vi "SPD.QEvsPow Meas Const T.vi"(5 "Continue":refnum<vi>, 6 "Temperature index":i32, 7 "Progress":refnum<vi>, 8 "Error In":errorcluster, 10 "TR_Bif Params":T1 {"scale type" items=["Linear", "Logarithmic"]}, 11 "SPD.Stand Ctrl in":T2={"spdDeviceSession"={"spdRef"=0, "connected"=FALSE, "spdName"="", "specification"={"diod case"=enum."default", "type"=enum."Unknown", "frequency"=enum."Unknown"}, "hidSPD.Controller"={"TSet"=0.0, "HV_bias"=0.0, "DDS_stb_code"=0}, "hidSPD.Sturtup Values"={"TSet"=0.0, "HV_bias"=0.0, "DDS_stb_code"=0}}, "DevBSession"={"DevBRef"="", "connected"=FALSE}, "FreqCSession"={"FreqCRef"="", "timeout"=0.0, "Gate"=0.0, "connected"=FALSE}, "8164BSession"={"Connection ID"=refnum, "Connected"=FALSE, "Info"="", "Slots Info"=[]}, "LeCroySession"={"LeCroySession"="", "connected"=FALSE}, "Events"={"DCRTest"=refnum, "Stop"=refnum}, "configFile"={"configFile ref"=refnum, "configFile path"=path "", "equipmentFile ref"=refnum}, "SPD.Meas Grid"={"DateTime"="", "DT"=[], "Insensitivity"=[], "Temprature"=[], "Stb_code"=[], "HV_Bias"=[]}, "SPD.Queues"={"state queue"=refnum}, "Console"=refnum} {"spdDeviceSession"."hidSPD.Sturtup Values"."HV_bias" format="%#_6p, V"; "spdDeviceSession"."hidSPD.Sturtup Values"."TSet" format="%#_6p, DegC"; "spdDeviceSession"."hidSPD.Controller"."HV_bias" format="%#_6p, V"; "spdDeviceSession"."hidSPD.Controller"."TSet" format="%#_6p, DegC"}) -> (0 "Error Out":errorcluster, 1 "pass":bool, 2 "Report":string, 3 "SPD.Stand Ctrl out":T2={"spdDeviceSession"={"spdRef"=0, "connected"=FALSE, "spdName"="", "specification"={"diod case"=enum."default", "type"=enum."Unknown", "frequency"=enum."Unknown"}, "hidSPD.Controller"={"TSet"=0.0, "HV_bias"=0.0, "DDS_stb_code"=0}, "hidSPD.Sturtup Values"={"TSet"=0.0, "HV_bias"=0.0, "DDS_stb_code"=0}}, "DevBSession"={"DevBRef"="", "connected"=FALSE}, "FreqCSession"={"FreqCRef"="", "timeout"=0.0, "Gate"=0.0, "connected"=FALSE}, "8164BSession"={"Connection ID"=refnum, "Connected"=FALSE, "Info"="", "Slots Info"=[]}, "LeCroySession"={"LeCroySession"="", "connected"=FALSE}, "Events"={"DCRTest"=refnum, "Stop"=refnum}, "configFile"={"configFile ref"=refnum, "configFile path"=path "", "equipmentFile ref"=refnum}, "SPD.Meas Grid"={"DateTime"="", "DT"=[], "Insensitivity"=[], "Temprature"=[], "Stb_code"=[], "HV_Bias"=[]}, "SPD.Queues"={"state queue"=refnum}, "Console"=refnum} {"spdDeviceSession"."hidSPD.Sturtup Values"."HV_bias" format="%#_6p, V"; "spdDeviceSession"."hidSPD.Sturtup Values"."TSet" format="%#_6p, DegC"; "spdDeviceSession"."hidSPD.Controller"."HV_bias" format="%#_6p, V"; "spdDeviceSession"."hidSPD.Controller"."TSet" format="%#_6p, DegC"})   [LabVIEW 2018]
uses:
  Instruments/KeySight 8164B/KeySight 8164B LAN InstrLib.lvlib
  typedefs/SPD.QE Strobe_Phase Tune Limits.ctl
  <vilib>/Analysis/NI_AALBase.lvlib
  <vilib>/Analysis/1siggen.llb/Ramp Pattern by Samples.vi
  Instruments/KC705 DevBoard/typedefs/DevB.Session.ctl
  Instruments/KeySight 53230A/typedefs/FreqC.Session.ctl
  Instruments/KeySight 8164B/KeySight 8164B LAN InstrLib/typedefs/KeySight 8164B control.ctl
  Instruments/LeCroy SDA830/typedefs/LeCroy.Session.ctl
  typedefs/SPD.Stand Ctrl.ctl
  typedefs/SPD.Events.ctl
  <vilib>/Utility/config.llb/Config Data RefNum.ctl
  <vilib>/Utility/config.llb/NI_LVConfig.lvlib
  typedefs/SPD.Meas Grid.ctl
  typedefs/SPD.Stand state.ctl
  typedefs/SPD.Queues.ctl
  ConfigFile/SPD.Config File ctrl.ctl
  Instruments/SPD HID Interface/hidSPDLibForLabView/LibVIs/hidSPD Controls/hidSPD Controller.ctl
  Instruments/SPD HID Interface/hidSPDLibForLabView/hidSPDLibForLabView.lvlib
  Instruments/SPD HID Interface/hidSPDLibForLabView/LibVIs/hidSPD Controls/hidSPD Device Session.ctl
  Instruments/SPD HID Interface/hidSPDLibForLabView/LibVIs/hidSPD Controls/hidSPD SPD Type.ctl
  typedefs/SPD.QEvsPower Test Params.ctl
  Instruments/SPD HID Interface/hidSPDLibForLabView/LibVIs/hidSPD Controls/hidSPD SPD Diod Case.ctl
  Instruments/SPD HID Interface/hidSPDLibForLabView/LibVIs/hidSPD Controls/hidSPD.STB Frequency.ctl
  Instruments/SPD HID Interface/hidSPDLibForLabView/LibVIs/hidSPD Controls/hidSPD.SPD specification.ctl
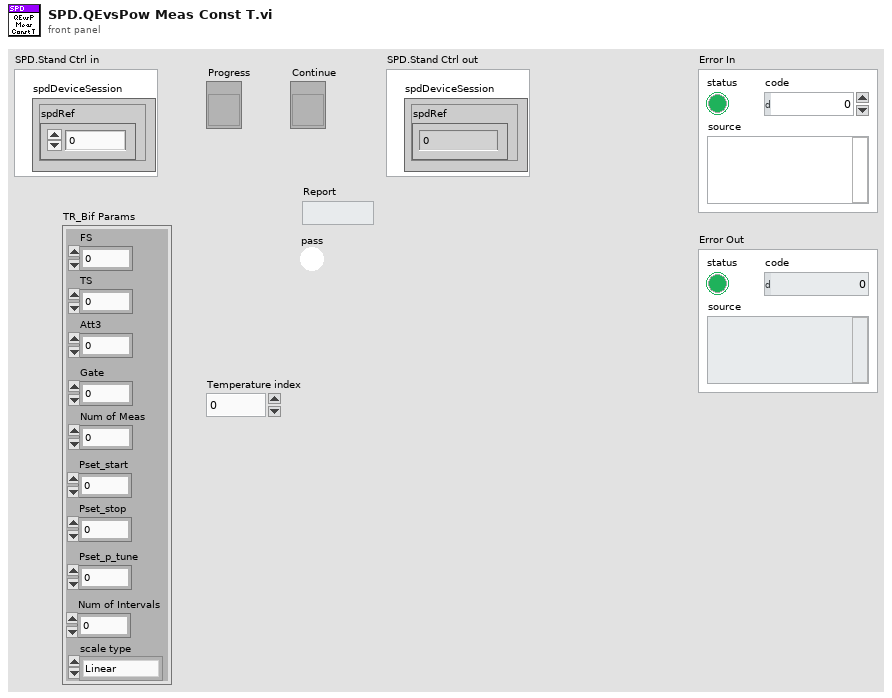
[diagram p1: front panel]
types:
  T1 = typedef "SPD.QEvsPower Test Params.ctl" = cluster{"FS":i32, "TS":i32, "Att3":dbl, "Gate":dbl, "Num of Meas":i32, "Pset_start":dbl, "Pset_p_tune":dbl, "Pset_stop":dbl, "Num of Intervals":i32, "scale type":u16}
  T2 = typedef "SPD.Stand Ctrl.ctl" = cluster{"spdDeviceSession":T3, "DevBSession":T9, "FreqCSession":T10, "8164BSession":T11, "LeCroySession":T12, "Events":T13, "configFile":T14, "SPD.Meas Grid":T16, "SPD.Queues":T17, "Console":refnum<vi>}
  T3 = typedef "hidSPDLibForLabView.lvlib/hidSPD Device Session.ctl" = cluster{"spdRef":u64, "connected":bool, "spdName":string, "specification":T4, "hidSPD.Controller":T8, "hidSPD.Sturtup Values":T8}
  T4 = typedef "hidSPDLibForLabView.lvlib/hidSPD.SPD specification.ctl" = cluster{"diod case":T5, "type":T6, "frequency":T7}
  T5 = typedef "hidSPDLibForLabView.lvlib/hidSPD SPD Diod Case.ctl" = enum16{"Unknown", "default", "butterfly"}
  T6 = typedef "hidSPDLibForLabView.lvlib/hidSPD SPD Type.ctl" = enum16{"Unknown", "Free Run", "Gate"}
  T7 = typedef "hidSPDLibForLabView.lvlib/hidSPD.STB Frequency.ctl" = enum16{"Unknown", "312", "1250"}
  T8 = typedef "hidSPDLibForLabView.lvlib/hidSPD Controller.ctl" = cluster{"TSet":sgl, "HV_bias":sgl, "DDS_stb_code":u16}
  T9 = typedef "DevB.Session.ctl" = cluster{"DevBRef":refnum<visa-resource-name>, "connected":bool}
  T10 = typedef "FreqC.Session.ctl" = cluster{"FreqCRef":refnum<visa-resource-name>, "timeout":dbl, "Gate":dbl, "connected":bool}
  T11 = typedef "KeySight 8164B LAN InstrLib.lvlib/KeySight 8164B control.ctl" = cluster{"Connection ID":refnum<k5>, "Connected":bool, "Info":string, "Slots Info":string[]}
  T12 = typedef "LeCroy.Session.ctl" = cluster{"LeCroySession":refnum<visa-resource-name>, "connected":bool}
  T13 = typedef "SPD.Events.ctl" = cluster{"DCRTest":refnum<user-event>, "Stop":refnum<user-event>}
  T14 = typedef "SPD.Config File ctrl.ctl" = cluster{"configFile ref":T15, "configFile path":path, "equipmentFile ref":T15}
  T15 = typedef "NI_LVConfig.lvlib/Config Data RefNum.ctl" = refnum<k1>
  T16 = typedef "SPD.Meas Grid.ctl" = cluster{"DateTime":string, "DT":dbl[], "Insensitivity":dbl[], "Temprature":dbl[], "Stb_code":dbl[], "HV_Bias":dbl[][][][]}
  T17 = typedef "SPD.Queues.ctl" = cluster{"state queue":refnum<queue>}
  T18 = typedef "SPD.QE Strobe_Phase Tune Limits.ctl" = cluster{"ph_start":i32, "ph_stop":i32, "ph_step":i32}
  T19 = typedef "hidSPDLibForLabView.lvlib/hidSPD SPD Type.ctl" = enum16{"Unknown", "Free Run", "Gate_312", "Gate_1250"}
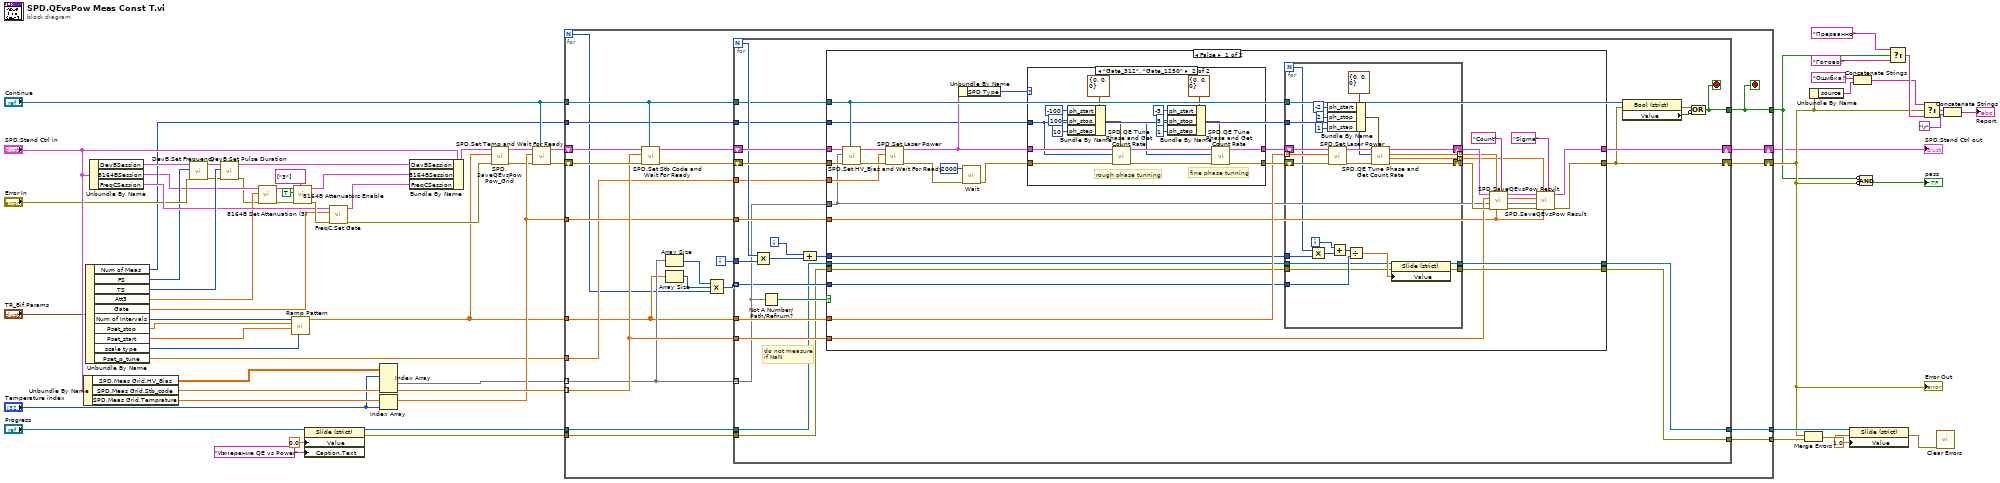
[diagram p0: block diagram]
diagram:
  n1 = Unbundle By Name("SPD.Stand Ctrl in") -> ("SPD.Meas Grid.HV_Bias"=w58:dbl[][][][], "SPD.Meas Grid.Stb_code"=w59:dbl[], "SPD.Meas Grid.Temprature"=w60:dbl[])
  n2 = Unbundle By Name("TR_Bif Params") -> ("Num of Meas"=w40:i32, "FS"=w38:i32, "TS"=w55:i32, "Att3"=w39:dbl, "Gate"=w41:dbl, "Num of Intervals"=w10:i32, "Pset_stop"=w9:dbl, "Pset_start"=w8:dbl, "scale type"=w6:u16, "Pset_p_tune"=w7:dbl)
  n3 = Unbundle By Name("SPD.Stand Ctrl in") -> ("DevBSession"=w57:T9, "8164BSession"=w12:T11, "FreqCSession"=w50:T10)
  n4 = call "DevB.Set Frequency.vi"("error in (no error)"="Error In", "Frequency"=w38, "DevB Session in"=w57) -> ("error out"=w54:errorcluster, "DevB Session out"=w56:T9)  [unwired: 7 in]
  n5 = call "DevB.Set Pulse Duration.vi"("error in (no error)"=w54, "Pulse Duration"=w55, "DevB Session in"=w56) -> ("error out"=w11:errorcluster, "DevB Session out"=w49:T9)  [unwired: 7 in]
  n6 = call "8164B Set Attenuation (3).vi"("error in"=w11, "Att 3, dB"=w39, "KeySight 8164B control in"=w12) -> ("error out"=w42:errorcluster, "KeySight 8164B control out"=w43:T11)  [unwired: 7 in]
  n7 = call-poly <vilib>:"Ramp Pattern.vi"("type"=w6, "start"=w8, "end"=w9, "samples"=w10) -> ("Ramp Pattern"=w1:dbl[])  [unwired: 6 in, 1 out]
  n8 = call "8164B Attenuators Enable.vi"("Slots"=string[] ["3"], "error in"=w42, "Enable"=TRUE, "KeySight 8164B control in"=w43) -> ("error out"=w51:errorcluster, "KeySight 8164B control out"=w48:T11)  [unwired: 6 in]
  n9 = property class="Slide (strict)"(reference="Progress", "Value"=0.0, "Caption.Text"="Измерение QE vs Power") -> (reference out=w18:refnum<vi>, error out=w16:errorcluster)  [unwired: 1 in]
  n10 = call "FreqC.Set Gate.vi"("error In"=w51, "Gate, sec"=w41, "FreqC Session in"=w50) -> ("error out"=w5:errorcluster, "FreqC Session out"=w47:T10)  [unwired: 7 in]
  n11 = Index Array(array=w58, index (dim 0)="Temperature index") -> (element=w21:dbl[][][])  [unwired: 3 in]
  n12 = Index Array(array=w60, index="Temperature index") -> (element=w22:dbl)
  n13 = Bundle By Name(cluster="SPD.Stand Ctrl in", "DevBSession"=w49, "8164BSession"=w48, "FreqCSession"=w47) -> (w3:T2)
  n14 = call "SPD.SaveQEvsPow Pow_Grid.vi"("Error In"=w5, "P_set_Grid"=w1, "SPD.Stand Ctrl in"=w3) -> ("Error Out"=w4:errorcluster, "SPD.Stand Ctrl out"=w2:T2)  [unwired: 7 in]
  n15 = call "SPD.Set Temp and Wait For Ready.vi"("Continue"="Continue", "Error In"=w4, "Tset"=w22, "SPD.Stand Ctrl in"=w2) -> ("Error Out"=w24:errorcluster, "SPD.Stand Ctrl out"=w23:T2)  [unwired: 6 in]
  n16 = for {
    N -> [w66]
    tunnel: w21 -> [w68] mode=indexing
    tunnel: w59 -> [w79] mode=indexing
    shift-right: [w87] -> w25
    shift-left: w23 -> [w85]
    shift-right: [w86] -> w28
    shift-left: w24 -> [w84]
    tunnel: "Continue" -> [w77]
    tunnel: [w82] -> w27
    tunnel: w18 -> [w81]
    tunnel: [w80] -> w63
    tunnel: w40 -> [w76]
    tunnel: w1 -> [w67]
    tunnel: w22 -> [w78]
    tunnel: w16 -> [w72]
    tunnel: [w71] -> w14
    tunnel: w7 -> [w69]
    i -> [w83]
    stop <- w82 stop-if-true
    n17 = call "SPD.Set Stb Code and Wait For Ready.vi"("Continue"=w77, "Error In"=w84, "Strobe code"=w79, "SPD.Stand Ctrl in"=w85) -> ("Error Out"=w74:errorcluster, "SPD.Stand Ctrl out"=w75:T2)  [unwired: 6 in]
    n18 = Array Size(array=w68) -> (size(s)=w70:i32[])
    n19 = Array Size(array=w67) -> (size(s)=w65:i32)
    n20 = Compound Arithmetic op=MULTIPLY(w70, w65, w66) -> (w73:i32[])
    n21 = for {
      N -> [w100]
      tunnel: w68 -> [w95] mode=indexing
      shift-right: [w103] -> w87
      shift-left: w75 -> [w112]
      shift-right: [w102] -> w86
      shift-left: w74 -> [w111]
      tunnel: w77 -> [w97]
      tunnel: w83 -> [w106]
      tunnel: [w108] -> w82
      tunnel: w81 -> [w91]
      tunnel: w73 -> [w92] mode=indexing
      tunnel: [w89] -> w80
      tunnel: w76 -> [w98]
      tunnel: w79 -> [w104]
      tunnel: w67 -> [w105]
      tunnel: w78 -> [w101]
      tunnel: w72 -> [w90]
      tunnel: [w88] -> w71
      tunnel: w69 -> [w94]
      i -> [w99]
      stop <- w108 stop-if-true
      # "do not measure\nif NaN"
      n22 = Multiply(x=w100, y=w106) -> (x*y=w107:i32)
      n23 = Not A Number/Path/Refnum?(number/path/refnum=w95) -> (NaN/Path/Refnum?=w96:bool[])
      n24 = Compound Arithmetic op=ADD(w99, w107) -> (w93:i32)
      n25 = case shown="False" w96 {
        tunnel: w112 -> [w146 w195]
        tunnel: w111 -> [w145 w194]
        tunnel: w105 -> [w134 _]
        tunnel: w104 -> [w117 _]
        tunnel: w95 -> [w116 _]
        tunnel: [w120 w195] -> w103
        tunnel: [w113 w194] -> w102
        tunnel: w101 -> [w115 _]
        tunnel: w98 -> [w132 _]
        tunnel: w97 -> [w133 _]
        tunnel: w94 -> [w137 _]
        tunnel: w93 -> [w128 _]
        tunnel: w92 -> [w127 _]
        tunnel: w91 -> [w126 w193]
        tunnel: w90 -> [w125 w192]
        tunnel: [w124 w193] -> w89
        tunnel: [w123 w192] -> w88
        frame False {
          n26 = call "SPD.Set HV_Bias and Wait For Ready.vi"("Continue"=w133, "Error In"=w145, "HV_Bias"=w116, "SPD.Stand Ctrl in"=w146) -> ("Error Out"=w140:errorcluster, "SPD.Stand Ctrl out"=w141:T2)  [unwired: 6 in]
          n27 = call "SPD.Set Laser Power.vi"("Error In"=w140, "Pset"=w137, "SPD.Stand Ctrl in"=w141) -> ("Error Out"=w138:errorcluster, "SPD.Stand Ctrl out"=w139:T2)  [unwired: 7 in]
          n28 = Unbundle By Name(w139) -> ("SPD Type"=w144:T19)
          n29 = call "Wait.vi"("error in (no error)"=w138, "milliseconds to wait"=u32 2000) -> ("error out"=w143:errorcluster)  [unwired: 9 in]
          n30 = case shown="\"Gate_312\", \"Gate_1250\"" w144 {
            tunnel: [w148 w160] -> w136
            tunnel: [w147 w159] -> w135
            tunnel: w139 -> [w148 w158]
            tunnel: w132 -> [_ w149]
            tunnel: w143 -> [w147 w150]
            frame "Free Run", Default {
            }
            frame "Gate_312", "Gate_1250" {
              # "fine phase tunning"
              # "rough phase tunning"
              n31 = Bundle By Name(cluster=T18 {"ph_start"=0, "ph_stop"=0, "ph_step"=0} ("SPD.QE Strobe_Phase Tune Limits"), "ph_start"=-100, "ph_stop"=100, "ph_step"=10) -> (w151:T18)
              n32 = call "SPD.QE Tune Phase and Get Count Rate.vi"("SPD.QE Strobe_Phase Tune Limits"=w151, "Error In"=w150, "Num of FreqC Meas"=w149, "SPD.Stand Ctrl in"=w158) -> ("Error Out"=w156:errorcluster, "SPD.Stand Ctrl out"=w157:T2)  [unwired: 4 in, 2 out]
              n33 = Bundle By Name(cluster=T18 {"ph_start"=0, "ph_stop"=0, "ph_step"=0} ("SPD.QE Strobe_Phase Tune Limits"), "ph_start"=-5, "ph_stop"=5, "ph_step"=1) -> (w164:T18)
              n34 = call "SPD.QE Tune Phase and Get Count Rate.vi"("SPD.QE Strobe_Phase Tune Limits"=w164, "Error In"=w156, "Num of FreqC Meas"=w149, "SPD.Stand Ctrl in"=w157) -> ("Error Out"=w159:errorcluster, "SPD.Stand Ctrl out"=w160:T2)  [unwired: 4 in, 2 out]
            }
          }
          n35 = for {
            N -> [w174]
            shift-right: [w180] -> w131
            shift-left: w136 -> [w191]
            shift-right: [w179] -> w130
            shift-left: w135 -> [w190]
            tunnel: w134 -> [w189] mode=indexing
            tunnel: w133 -> [_]
            tunnel: w132 -> [w181]
            tunnel: [w178] -> w129 mode=indexing
            tunnel: [w177] -> w119 mode=indexing
            tunnel: w128 -> [w175]
            tunnel: w127 -> [w170]
            tunnel: w126 -> [w169]
            tunnel: w125 -> [w168]
            tunnel: [w167] -> w124
            tunnel: [w166] -> w123
            i -> [w172]
            n36 = Multiply(x=w174, y=w175) -> (x*y=w173:i32)
            n37 = Bundle By Name(cluster=T18 {"ph_start"=0, "ph_stop"=0, "ph_step"=0} ("SPD.QE Strobe_Phase Tune Limits"), "ph_start"=-2, "ph_stop"=2, "ph_step"=1) -> (w187:T18)
            n38 = call "SPD.Set Laser Power.vi"("Error In"=w190, "Pset"=w189, "SPD.Stand Ctrl in"=w191) -> ("Error Out"=w182:errorcluster, "SPD.Stand Ctrl out"=w183:T2)  [unwired: 7 in]
            n39 = Add(x=w172, y=w173) -> (x+y=w171:i32)
            n40 = Divide(x=w171, y=w170) -> (x/y=w176:dbl)
            n41 = call "SPD.QE Tune Phase and Get Count Rate.vi"("SPD.QE Strobe_Phase Tune Limits"=w187, "Error In"=w182, "Num of FreqC Meas"=w181, "SPD.Stand Ctrl in"=w183) -> ("Error Out"=w179:errorcluster, "Count Sigma"=w177:dbl, "Count Rate"=w178:dbl, "SPD.Stand Ctrl out"=w180:T2)  [unwired: 4 in]
            n42 = property class="Slide (strict)"(reference=w169, error in=w168, "Value"=w176) -> (reference out=w167:refnum<vi>, error out=w166:errorcluster)
          }
          n43 = call "SPD.SaveQEvsPow Result.vi"("result name"="Count", "Temperature"=w115, "result"=w129, "Error In"=w130, "HV_bias"=w116, "Stb_Code"=w117, "SPD.Stand Ctrl in"=w131) -> ("Error Out"=w114:errorcluster, "SPD.Stand Ctrl out"=w121:T2)  [unwired: 3 in]
          n44 = call "SPD.SaveQEvsPow Result.vi"("result name"="Sigma", "Temperature"=w115, "result"=w119, "Error In"=w114, "HV_bias"=w116, "Stb_Code"=w117, "SPD.Stand Ctrl in"=w121) -> ("Error Out"=w113:errorcluster, "SPD.Stand Ctrl out"=w120:T2)  [unwired: 3 in]
        }
        frame True {
        }
      }
      n45 = property class="Bool (strict)"(reference=w97, error in=w102) -> (error out=w109:errorcluster, "Value"=w110:bool)  [unwired: 1 out]
      n46 = Compound Arithmetic op=OR(w109, invert w110) -> (w108:bool)
    }
  }
  "SPD.Stand Ctrl out" <- w25
  "Error Out" <- w28
  n47 = Merge Errors(w28, w14) -> (w15:errorcluster)
  n48 = Unbundle By Name(w28) -> ("source"=w33:string)
  n49 = property class="Slide (strict)"(reference=w63, error in=w15, "Value"=1.0) -> (error out=w61:errorcluster)  [unwired: 1 out]
  n50 = Concatenate Strings("Ошибка!" ("t"), w33) -> (w34:string)
  n51 = Compound Arithmetic op=AND(invert w27, invert w28) -> (→"pass":bool)
  n52 = Select(t="Прерванно" ("Report"), s=w27, f="Готово!") -> (s? t:f=w36:string)
  n53 = Select(t=w34, s=w28, f=w36) -> (s? t:f=w31:string)
  n54 = call <vilib>:"Clear Errors.vi"("error in (no error)"=w61) -> ()  [unwired: 5 in, 2 out]
  n55 = Concatenate Strings(w31, "\r") -> (→"Report":string)
